vi "LUT.vi"() -> ()   [LabVIEW 2010]
uses:
  <vilib>/Utility/file.llb/Read From Spreadsheet File (string).vi
panel:
  out "Lookup Result:":string[][](array[string])
  out "Status:":string
  in  "stop":bool
  in  "Lookup:":T1
  out "LUT:":string[][](array[string])
  in  "LUT File":path=path "C:/Users/schalla/Desktop/LUT/LUT.csv"
  # "Param 1"
  # "Param 2"
  # "Param 3"
  # "Use?"
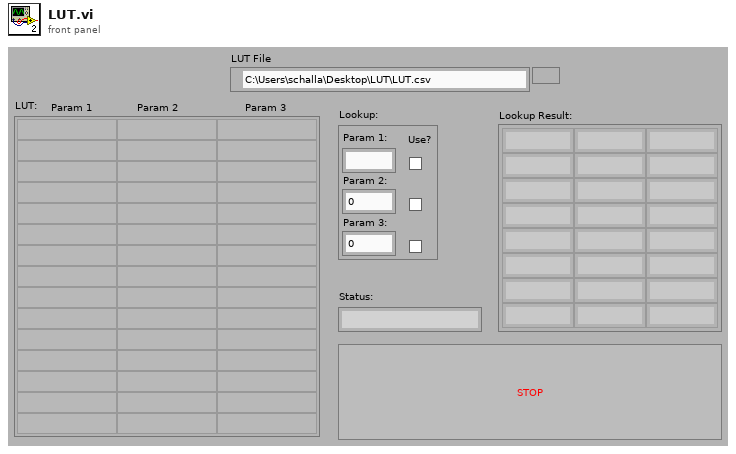
[diagram p1: front panel]
types:
  T1 = cluster{"Param 1:":string, "Param 2:":dbl, "Param 3:":dbl, "1":bool, "2":bool, "3":bool}
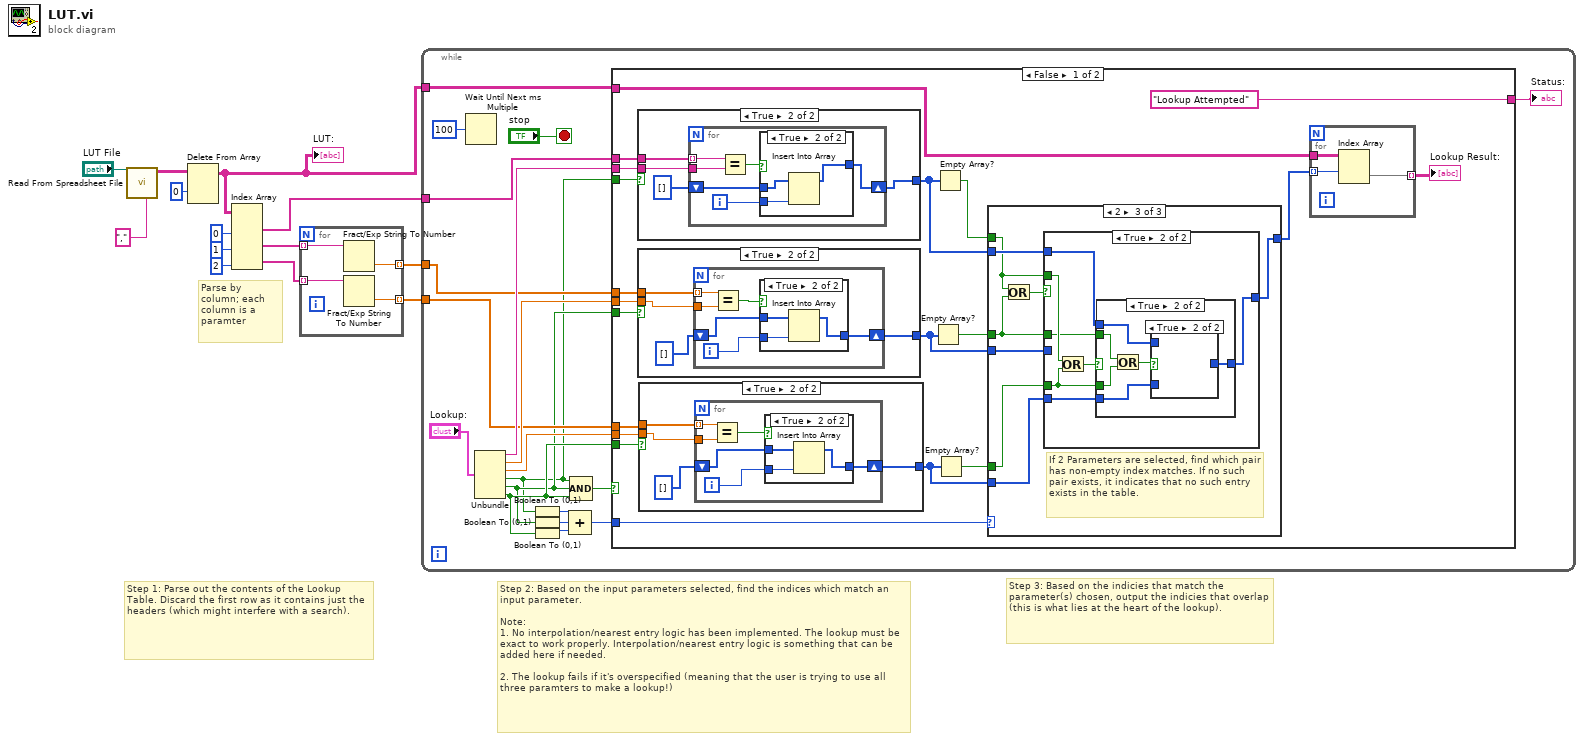
[diagram p0: block diagram]
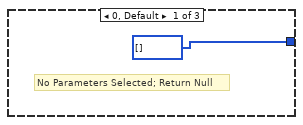
[diagram p2: hidden frame]
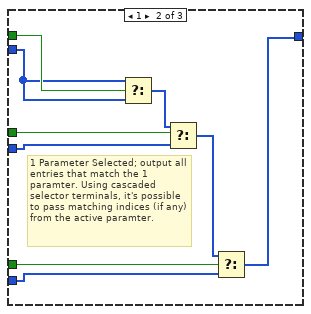
[diagram p3: hidden frame]
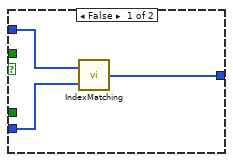
[diagram p4: hidden frame]
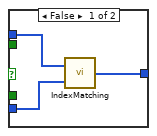
[diagram p5: hidden frame]
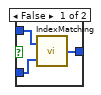
[diagram p6: hidden frame]
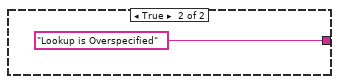
[diagram p13: hidden frame]
diagram:
  # "Parse by column; each column is a  paramter"
  # "Step 3: Based on the indicies that match the parameter(s) chosen, output the indicies that overlap (this is what lies at the heart of the lookup)."
  # "Step 2: Based on the input parameters selected, find the indices which match an input parameter.\n\nNote: \n1. No interpolation/nearest entry logic has been implemented. The lookup must be exact to work properly. Interpolation/nearest entry logic is something that can be added here if needed.\n\n2. The lookup fails if it's overspecified (meaning that the user is trying to use all three paramters to make a lookup!)"
  # "Step 1: Parse out the contents of the Lookup Table. Discard the first row as it contains just the headers (which might interfere with a search)."
  n1 = call-poly <vilib>:"Read From Spreadsheet File.vi"("delimiter (\\t)"="," ("delimiter (\\t)"), "file path (dialog if empty)"="LUT File") -> ("all rows"=w4:string[][])  [unwired: 5 in, 4 out]
  n2 = Delete From Array(array=w4, index (row)=0) -> (array with subset deleted=w2:string[][])  [unwired: 2 in, 1 out]
  "LUT:" <- w2
  n3 = Index Array(array=w2, index (col) #1=0 ("disabled index (col)"), index (col) #2=1 ("index (col)"), index (col) #3=2 ("index (col)")) -> (element #1=w1:string[], element #2=w5:string[], element #3=w8:string[])  [unwired: 3 in]
  n4 = for {
    tunnel: w8 -> [w17] mode=indexing
    tunnel: [w16] -> w7 mode=indexing
    tunnel: [w15] -> w6 mode=indexing
    tunnel: w5 -> [w14] mode=indexing
    n5 = Fract/Exp String To Number(string=w14) -> (number=w16:dbl)  [unwired: 3 in, 1 out]
    n6 = Fract/Exp String To Number(string=w17) -> (number=w15:dbl)  [unwired: 3 in, 1 out]
  }
  n7 = while {
    tunnel: w1 -> [w33]
    tunnel: w7 -> [w31]
    tunnel: w6 -> [w29]
    tunnel: w2 -> [w27]
    stop <- "stop" stop-if-true
    n8 = Wait Until Next ms Multiple(millisecond multiple=u32 100) -> ()  [unwired: 1 out]
    n9 = Unbundle("Lookup:") -> ("Param 1:"=w32:string, "Param 2:"=w30:dbl, "Param 3:"=w28:dbl, "1"=w24:bool, "2"=w25:bool, "3"=w26:bool)
    n10 = Boolean To (0,1)(Boolean=w24) -> (0, 1=w22:i16)
    n11 = Boolean To (0,1)(Boolean=w25) -> (0, 1=w21:i16)
    n12 = Boolean To (0,1)(Boolean=w26) -> (0, 1=w20:i16)
    n13 = Compound Arithmetic op=ADD(w22, w21, w20) -> (w19:i16)
    n14 = Compound Arithmetic op=AND(w24, w25, w26) -> (w23:bool)
    n15 = case shown="False" w23 {
      tunnel: ["Lookup Attempted" ("t") "Lookup is Overspecified" ("t")] -> w34
      tunnel: w33 -> [w47 _]
      tunnel: w32 -> [w48 _]
      tunnel: w24 -> [w55 _]
      tunnel: w31 -> [w51 _]
      tunnel: w30 -> [w52 _]
      tunnel: w25 -> [w54 _]
      tunnel: w29 -> [w49 _]
      tunnel: w28 -> [w50 _]
      tunnel: w26 -> [w53 _]
      tunnel: w27 -> [w46 _]
      tunnel: w19 -> [w44 _]
      frame False {
        n16 = case shown="True" w55 {
          tunnel: w48 -> [_ w131]
          tunnel: w47 -> [_ w130]
          tunnel: [_ w128] -> w43
          frame False {
          }
          frame True {
            n17 = for {
              tunnel: w131 -> [w137]
              tunnel: w130 -> [w136] mode=indexing
              shift-right: [w132] -> w128
              shift-left: i32[] [] -> [w134]
              i -> [w133]
              n18 = Equal?(x=w136, y=w137) -> (x = y?=w135:bool)
              n19 = case shown="True" w135 {
                tunnel: w134 -> [w138 w141]
                tunnel: w133 -> [_ w139]
                tunnel: [w138 w140] -> w132
                frame False {
                }
                frame True {
                  n20 = Insert Into Array(array=w141, new element=w139) -> (w140:i32[])  [unwired: 1 in]
                }
              }
            }
          }
        }
        n21 = case shown="True" w54 {
          tunnel: w52 -> [_ w114]
          tunnel: w51 -> [_ w115]
          tunnel: [_ w116] -> w40
          frame False {
          }
          frame True {
            n22 = for {
              tunnel: w115 -> [w122] mode=indexing
              tunnel: w114 -> [w123]
              shift-right: [w118] -> w116
              shift-left: i32[] [] -> [w120]
              i -> [w119]
              n23 = Equal?(x=w122, y=w123) -> (x = y?=w121:bool)
              n24 = case shown="True" w121 {
                tunnel: w120 -> [w124 w127]
                tunnel: w119 -> [_ w126]
                tunnel: [w124 w125] -> w118
                frame False {
                }
                frame True {
                  n25 = Insert Into Array(array=w127, new element=w126) -> (w125:i32[])  [unwired: 1 in]
                }
              }
            }
          }
        }
        n26 = case shown="True" w53 {
          tunnel: w50 -> [_ w100]
          tunnel: w49 -> [_ w101]
          tunnel: [_ w102] -> w38
          frame False {
          }
          frame True {
            n27 = for {
              tunnel: w101 -> [w108] mode=indexing
              tunnel: w100 -> [w109]
              shift-right: [w104] -> w102
              shift-left: i32[] [] -> [w106]
              i -> [w105]
              n28 = Equal?(x=w108, y=w109) -> (x = y?=w107:bool)
              n29 = case shown="True" w107 {
                tunnel: w106 -> [w110 w113]
                tunnel: w105 -> [_ w112]
                tunnel: [w110 w111] -> w104
                frame False {
                }
                frame True {
                  n30 = Insert Into Array(array=w113, new element=w112) -> (w111:i32[])  [unwired: 1 in]
                }
              }
            }
          }
        }
        n31 = Empty Array?(array=w40) -> (empty?=w41:bool)
        n32 = Empty Array?(array=w43) -> (empty?=w42:bool)
        n33 = Empty Array?(array=w38) -> (empty?=w39:bool)
        n34 = case shown="2" w44 {
          tunnel: w43 -> [_ w65 w73]
          tunnel: w42 -> [_ w66 w70]
          tunnel: w41 -> [_ w64 w67]
          tunnel: w40 -> [_ w62 w72]
          tunnel: w39 -> [_ w61 w69]
          tunnel: w38 -> [_ w60 w68]
          tunnel: [i32[] [] w58 w71] -> w37
          frame 0, Default {
            # "No Parameters Selected; Return Null"
          }
          frame 1 {
            # "1 Parameter Selected; output all entries that match the 1 paramter. Using cascaded selector terminals, it's possible to pass matching indices (if any) from the active paramter."
            n35 = Select(t=w65, s=w66, f=w65) -> (s? t:f=w63:i32[])
            n36 = Select(t=w63, s=w64, f=w62) -> (s? t:f=w59:i32[])
            n37 = Select(t=w59, s=w61, f=w60) -> (s? t:f=w58:i32[])
          }
          frame 2 {
            # "If 2 Parameters are selected, find which pair has non-empty index matches. If no such pair exists, it indicates that no such entry exists in the table."
            n38 = Or(x=w70, y=w67) -> (x .or. y?=w74:bool)
            n39 = case shown="True" w74 {
              tunnel: w73 -> [w77 w81]
              tunnel: w72 -> [w76 _]
              tunnel: [w75 w80] -> w71
              tunnel: w70 -> [_ w84]
              tunnel: w69 -> [_ w78]
              tunnel: w68 -> [_ w82]
              tunnel: w67 -> [_ w79]
              frame False {
                n40 = call "IndexMatching.vi"("Array2"=w76, "Array1"=w77) -> ("Matched Indices"=w75:i32[])
              }
              frame True {
                n41 = Or(x=w84, y=w78) -> (x .or. y?=w83:bool)
                n42 = case shown="True" w83 {
                  tunnel: w82 -> [w87 w89]
                  tunnel: w81 -> [w86 w88]
                  tunnel: [w85 w90] -> w80
                  tunnel: w79 -> [_ w93]
                  tunnel: w78 -> [_ w92]
                  frame False {
                    n43 = call "IndexMatching.vi"("Array2"=w87, "Array1"=w86) -> ("Matched Indices"=w85:i32[])
                  }
                  frame True {
                    n44 = Or(x=w93, y=w92) -> (x .or. y?=w91:bool)
                    n45 = case shown="True" w91 {
                      tunnel: [w96 _] -> w90
                      tunnel: w89 -> [w95 _]
                      tunnel: w88 -> [w94 _]
                      frame False {
                        n46 = call "IndexMatching.vi"("Array2"=w95, "Array1"=w94) -> ("Matched Indices"=w96:i32[])
                      }
                      frame True {
                      }
                    }
                  }
                }
              }
            }
          }
        }
        n47 = for {
          tunnel: [w99] -> w45 mode=indexing
          tunnel: w46 -> [w98]
          tunnel: w37 -> [w97] mode=indexing
          n48 = Index Array(array=w98, index (row)=w97) -> (element=w99:string[])  [unwired: 1 in]
        }
        "Lookup Result:" <- w45
      }
      frame True {
      }
    }
    "Status:" <- w34
  }
